vi "题目2.vi"() -> ()   [LabVIEW 2017]
panel:
  out "数值 2":dbl
  out "数值":dbl
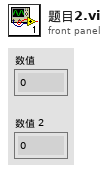
[diagram p1: front panel]
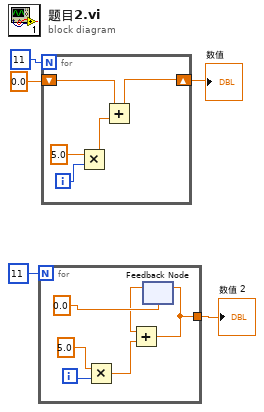
[diagram p0: block diagram]
diagram:
  n1 = for {
    N: 11 -> [_]
    tunnel: [w8] -> w1
    i -> [w11]
    n2 = Multiply(x=5.0, y=w11) -> (x*y=w7:dbl)
    n3 = feedback #1(0.0) -> (w9:dbl)
    n4 = Add(x=w9, y=w7) -> (x+y=w8:dbl)
    n5 = feedback-in #1(w8) -> ()
  }
  "数值 2" <- w1
  n6 = for {
    N: 11 -> [_]
    shift-right: [w12] -> w3
    shift-left: 0.0 -> [w13]
    i -> [w15]
    n7 = Multiply(x=5.0, y=w15) -> (x*y=w14:dbl)
    n8 = Add(x=w13, y=w14) -> (x+y=w12:dbl)
  }
  "数值" <- w3
